vi "TagDB-Delete Multiple.vi"(8 "error in (no error)":errorcluster, 10 "Tags":string[](array[string]), 11 "TagDB":T1) -> (0 "error out":errorcluster, 3 "TagDB(dup)":T1)   [LabVIEW 2017, in "TagDB.lvlib"]
uses:
  TagDB.lvlib
  Typedef/TagDB.ctl
  _Support/Error/_Build Error Cluster.vi
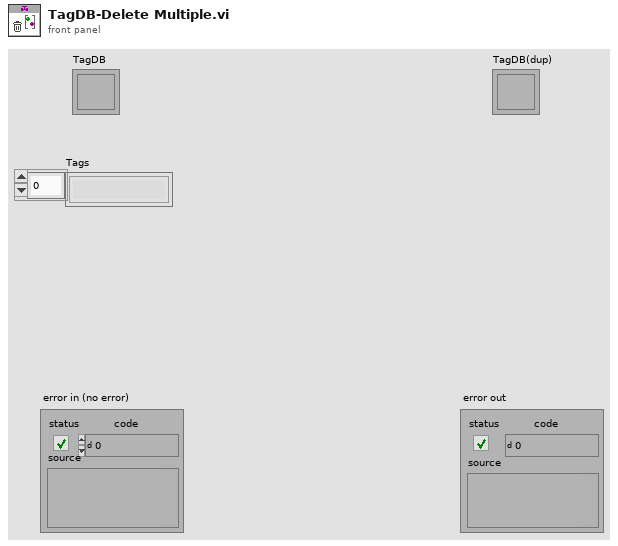
[diagram p1: front panel]
types:
  T1 = typedef "TagDB.lvlib/TagDB.ctl" = refnum<k1>
  T2 = typedef "TagDB.lvlib/tagdb-data.ctl" = cluster{"tag-map":variant, "timestamp-map":variant, "namecacher-map":variant, "DataTypeCacher-map":variant, "Tag Adding Lock?":bool, "Global Change Timestamp":timestamp, "Item Change Timestamp":timestamp, "name":string, "Global Change Flag":u64, "Item Change Flag":u64}
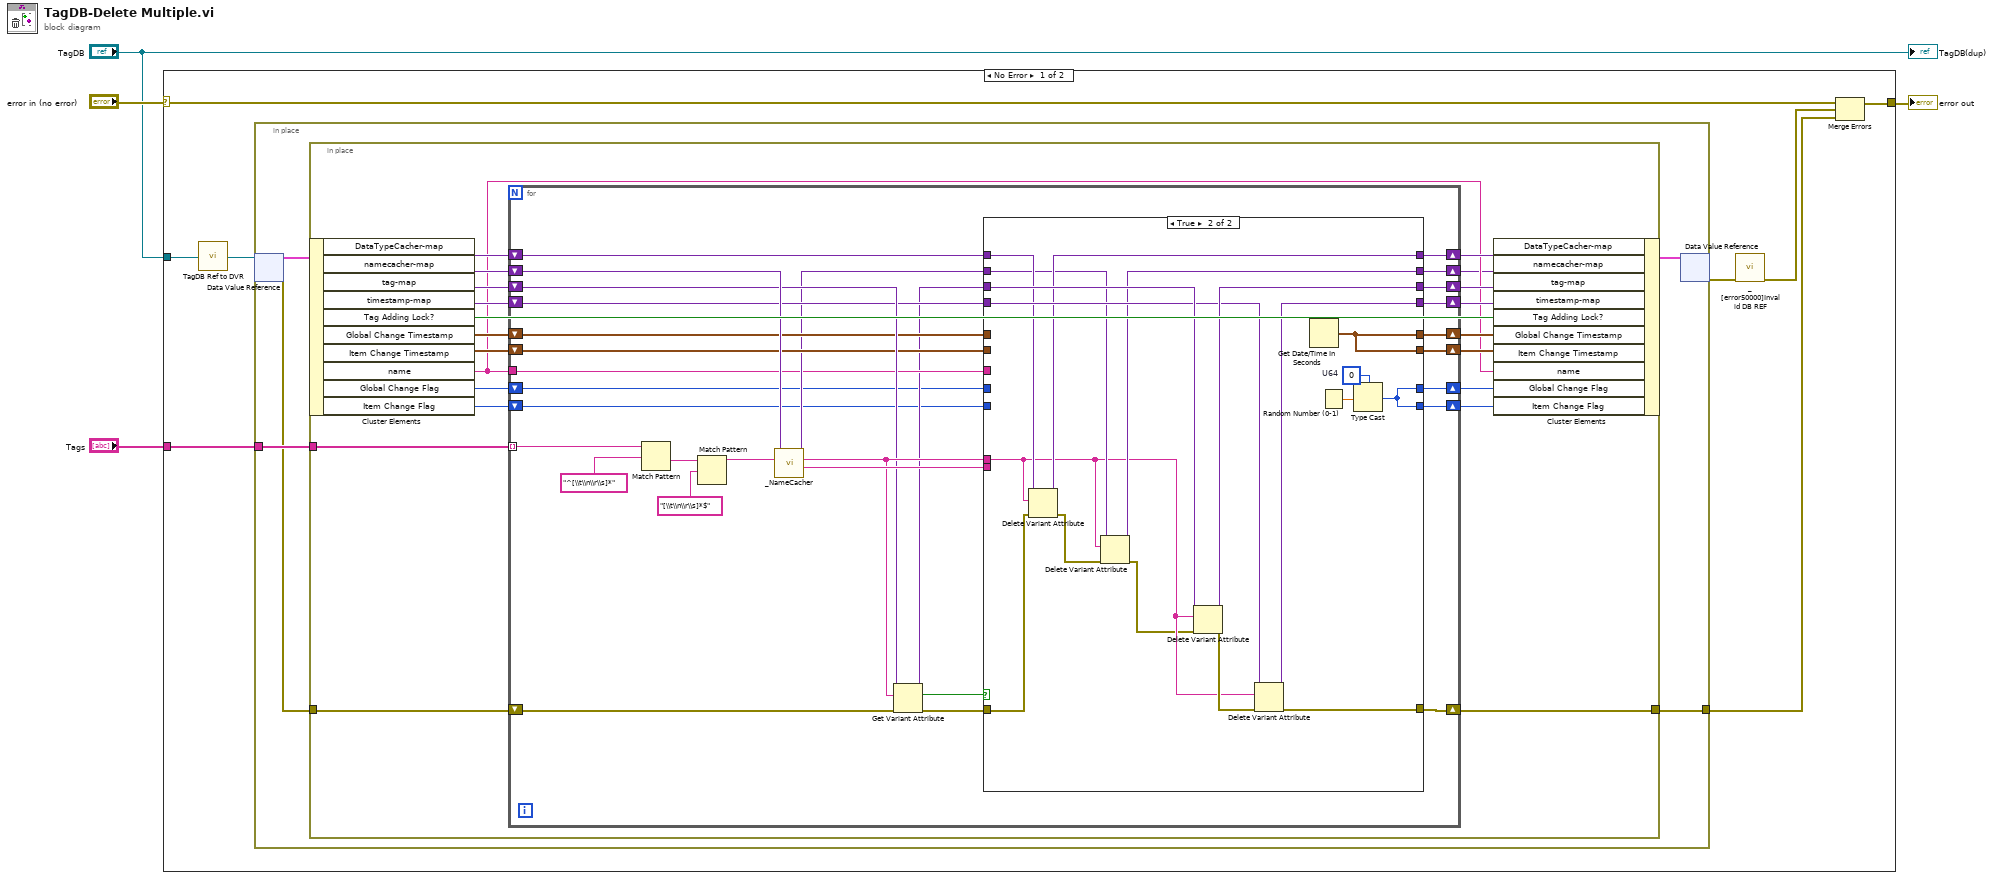
[diagram p0: block diagram]
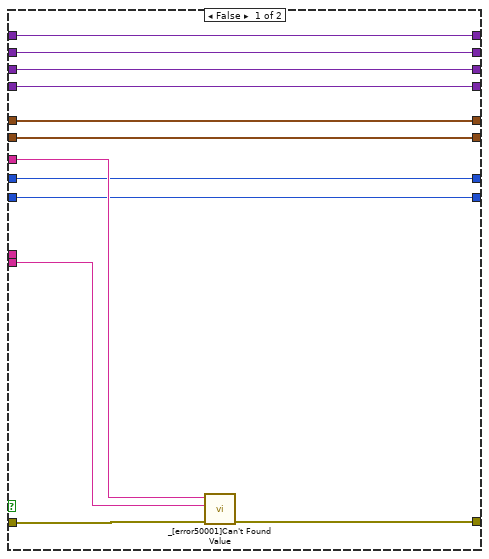
[diagram p2: hidden frame]
diagram:
  n1 = case shown="No Error" "error in (no error)" {
    selector: "error in (no error)" -> [w10 w99]
    tunnel: [w11 w99] -> w3
    tunnel: "TagDB" -> [w8 _]
    tunnel: "Tags" -> [w6 _]
    frame No Error {
      n2 = call "TagDB Ref to DVR.vi"("TagDB"=w8) -> ("DVR"=w7:refnum<data-value>)  [unwired: 4 in]
      n3 = in-place "In Place Element Structure" {
        in-place-border: [w17] -> w12
        in-place-border: w6 -> [w16]
        n4 = in-place-dvr #1(w7) -> (w15:T2, w13:errorcluster)
        n5 = in-place {
          in-place-border: [w38] -> w17
          in-place-border: w16 -> [w18]
          in-place-border: w13 -> [w32]
          n6 = in-place-cluster #2(w15) -> ("DataTypeCacher-map"=w25:variant, "namecacher-map"=w37:variant, "tag-map"=w36:variant, "timestamp-map"=w35:variant, "Tag Adding Lock?"=w29:bool, "Global Change Timestamp"=w31:timestamp, "Item Change Timestamp"=w28:timestamp, "name"=w24:string, "Global Change Flag"=w21:u64, "Item Change Flag"=w20:u64)
          n7 = for {
            tunnel: w24 -> [w51]
            tunnel: w18 -> [w40] mode=indexing
            shift-right: [w53] -> w23
            shift-left: w37 -> [w65]
            shift-right: [w62] -> w34
            shift-left: w36 -> [w64]
            shift-right: [w61] -> w33
            shift-left: w35 -> [w63]
            shift-right: [w68] -> w38
            shift-left: w32 -> [w60]
            shift-right: [w58] -> w30
            shift-left: w31 -> [w59]
            shift-right: [w56] -> w27
            shift-left: w28 -> [w57]
            shift-right: [w55] -> w26
            shift-left: w25 -> [w54]
            shift-right: [w47] -> w22
            shift-left: w21 -> [w46]
            shift-right: [w44] -> w19
            shift-left: w20 -> [w45]
            n8 = Match Pattern(string=w40, regular expression="^[\\t\\n\\r\\s]*") -> (after substring=w41:string)  [unwired: 1 in, 3 out]
            n9 = Match Pattern(string=w41, regular expression="[\\t\\n\\r\\s]*$") -> (before substring=w39:string)  [unwired: 1 in, 3 out]
            n10 = call "_NameCacher.vi"("key"=w39, "cacher"=w65) -> ("Raw name"=w67:string, "Key in lower case"=w66:string, "cacher out"=w52:variant)  [unwired: 7 in]
            n11 = Get Variant Attribute(Variant=w64, name=w66, error in=w60) -> (duplicate Variant=w49:variant, found=w48:bool, error out=w50:errorcluster)  [unwired: 1 in, 1 out]
            n12 = case shown="True" w48 {
              tunnel: [w73 w97] -> w68
              tunnel: w67 -> [w72 _]
              tunnel: w50 -> [w74 w84]
              tunnel: w49 -> [w80 w96]
              tunnel: [w80 w95] -> w62
              tunnel: w63 -> [w79 w93]
              tunnel: [w79 w94] -> w61
              tunnel: w66 -> [_ w87]
              tunnel: [w78 w92] -> w58
              tunnel: w59 -> [w78 _]
              tunnel: [w77 w92] -> w56
              tunnel: w57 -> [w77 _]
              tunnel: [w76 w90] -> w55
              tunnel: w54 -> [w76 w91]
              tunnel: [w75 w88] -> w53
              tunnel: w52 -> [w75 w89]
              tunnel: w51 -> [w71 _]
              tunnel: [w70 w81] -> w47
              tunnel: w46 -> [w70 _]
              tunnel: w45 -> [w69 _]
              tunnel: [w69 w81] -> w44
              frame False {
                n13 = call "_[error50001]Can't Found Value.vi"("error in (no error)"=w74, "db name"=w72, "value name"=w71) -> ("error out"=w73:errorcluster)  [unwired: 8 in]
              }
              frame True {
                w82 = u64 0  # U64
                n14 = Delete Variant Attribute(4:w84, 6:w87, 7:w91) -> (0:w86:errorcluster, 3:w90:variant)  [unwired: 1 out]
                n15 = Delete Variant Attribute(4:w86, 6:w87, 7:w89) -> (0:w85:errorcluster, 3:w88:variant)  [unwired: 1 out]
                n16 = Delete Variant Attribute(4:w85, 6:w87, 7:w96) -> (0:w98:errorcluster, 3:w95:variant)  [unwired: 1 out]
                n17 = Delete Variant Attribute(4:w98, 6:w87, 7:w93) -> (0:w97:errorcluster, 3:w94:variant)  [unwired: 1 out]
                n18 = Get Date/Time In Seconds() -> (seconds since 1Jan1904=w92:timestamp)
                n19 = Random Number (0-1)() -> (number: 0 to 1=w83:dbl)
                n20 = Type Cast(type=w82, x=w83) -> (*(type *) &x=w81:u64)
              }
            }
          }
          n21 = in-place-cluster #2("DataTypeCacher-map"=w26, "namecacher-map"=w23, "tag-map"=w34, "timestamp-map"=w33, "Tag Adding Lock?"=w29, "Global Change Timestamp"=w30, "Item Change Timestamp"=w27, "name"=w24, "Global Change Flag"=w22, "Item Change Flag"=w19) -> (w14:T2)
        }
        n22 = in-place-dvr #1(w14) -> (w9:errorcluster)  [unwired: 1 out]
      }
      n23 = call "_[error50000]Invalid DB REF.vi"("error in (no error)"=w9) -> ("error out"=w5:errorcluster)  [unwired: 10 in]
      n24 = Merge Errors(w10, w5, w12) -> (w11:errorcluster)
    }
    frame Error {
    }
  }
  "error out" <- w3
  "TagDB(dup)" <- "TagDB"
